vi "Apply Desired to Imported Data.vi"(0 "table.Data In":string[][](array[string]), 7 "StatArray":string[][](array[string]), 9 "Controller":T3, 11 "Stability Cluster":T4) -> (4 "table.Data Out":string[][](array[string]), 15 "StatBundle Out":T1(array[cluster]))   [LabVIEW 2013]
uses:
  TypeDef/Stability Cluster.ctl
  TypeDef/Controller Names.ctl
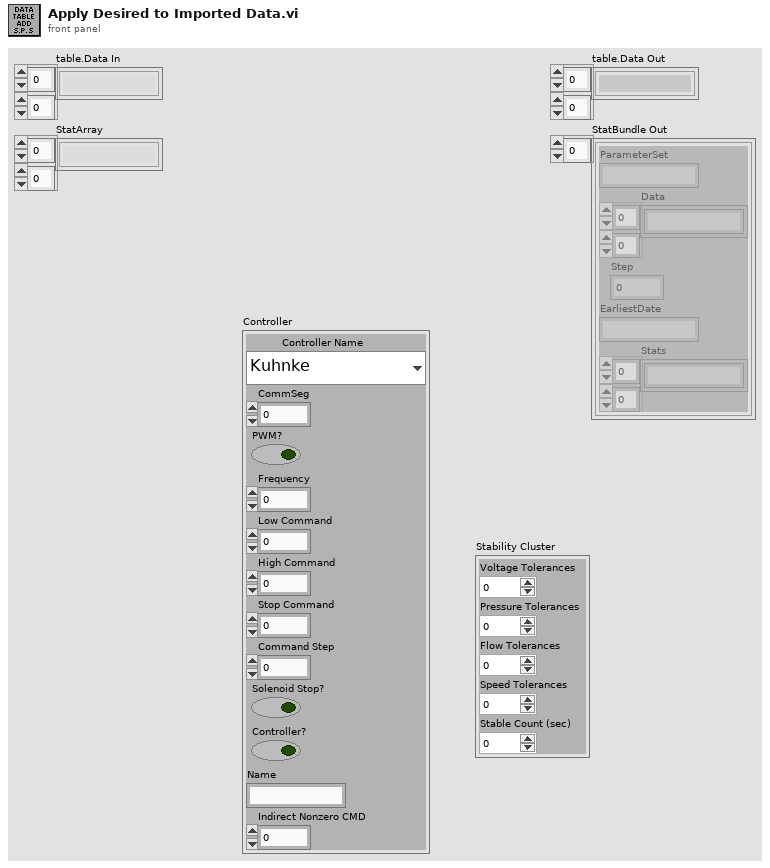
[diagram p1: front panel]
types:
  T1 = cluster{"ParameterSet":string, "Data":string[][], "Step":i32, "EarliestDate":string, "Stats":string[][]}[]
  T2 = typedef "Controller Names.ctl" = enum16{"Kuhnke", "McLaren", "Helbako BLDC", "Conti", "Hella E4LMF", "Hella E4LMD", "Hella E4DCG 20mm", "Hella E4DCG 30mm", "Helbako (old)", "TI PWM", "PSA", "Hella Hyundai Gas", "Hella Hyundai Diesel", "8 Comm", "10 Comm", "8 Comm Hella FCA", "10 Comm Hella FCA", "8 Comm Omron", "10 Comm Omron", "8 Comm Nissan", "10 Comm Nissan"}
  T3 = cluster{"Controller Name":T2, "CommSeg":i32, "PWM?":bool, "Frequency":i32, "Low Command":dbl, "High Command":dbl, "Stop Command":dbl, "Command Step":dbl, "Solenoid Stop?":bool, "Controller?":bool, "Name":string, "Indirect Nonzero CMD":dbl}
  T4 = typedef "Stability Cluster.ctl" = cluster{"Voltage Tolerances":dbl, "Pressure Tolerances":dbl, "Flow Tolerances":dbl, "Speed Tolerances":dbl, "Stable Count (sec)":dbl}
  T5 = typedef "Command Cluster.ctl" = cluster{"Para1":i32, "SP1":dbl, "Para2":i32, "SP2":dbl, "Para3":i32, "SP3":dbl}
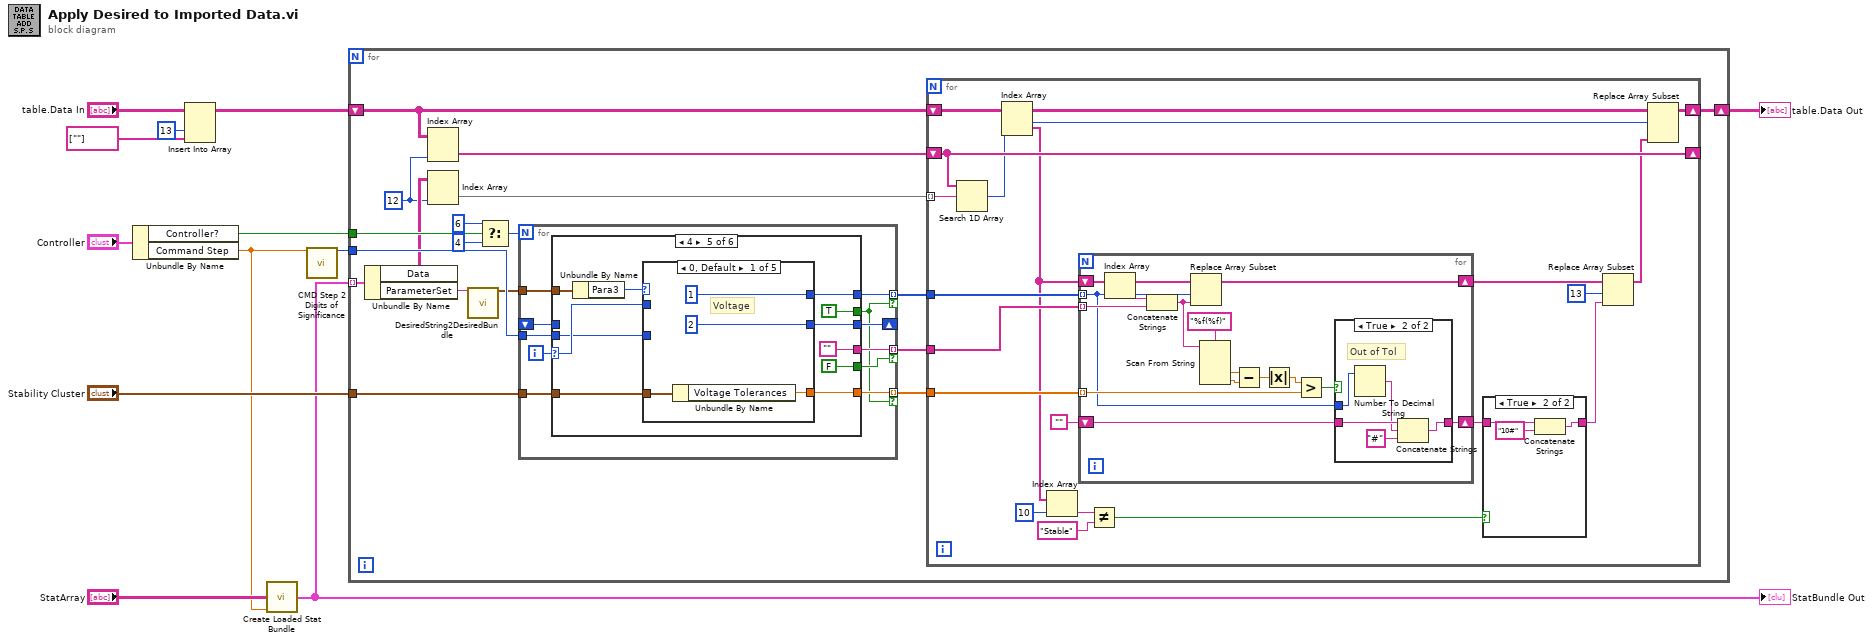
[diagram p0: block diagram]
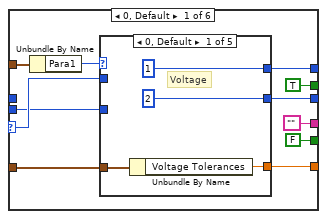
[diagram p4: hidden frame]
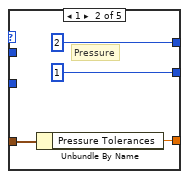
[diagram p5: hidden frame]
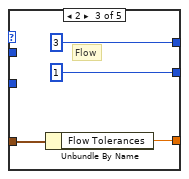
[diagram p6: hidden frame]
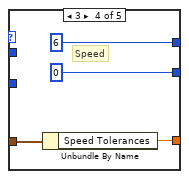
[diagram p7: hidden frame]
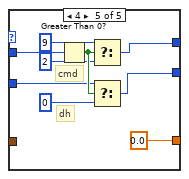
[diagram p8: hidden frame]
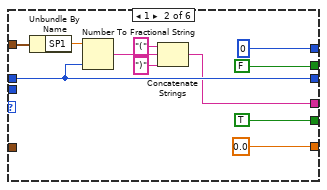
[diagram p9: hidden frame]
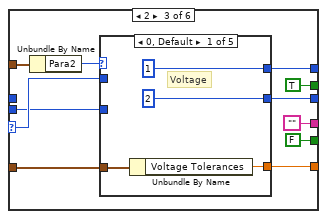
[diagram p10: hidden frame]
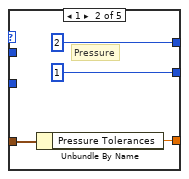
[diagram p11: hidden frame]
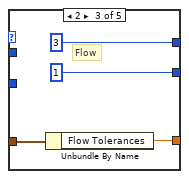
[diagram p12: hidden frame]
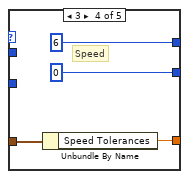
[diagram p13: hidden frame]
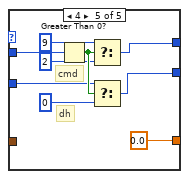
[diagram p14: hidden frame]
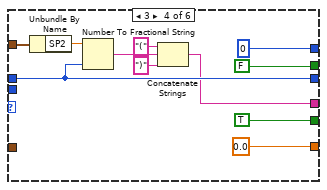
[diagram p15: hidden frame]
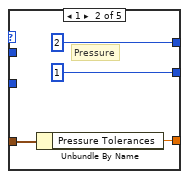
[diagram p16: hidden frame]
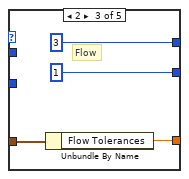
[diagram p17: hidden frame]
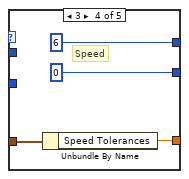
[diagram p18: hidden frame]
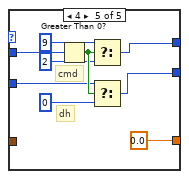
[diagram p19: hidden frame]
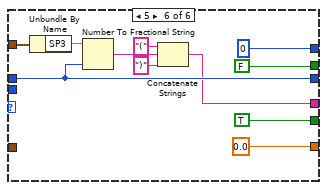
[diagram p20: hidden frame]
diagram:
  n1 = Unbundle By Name("Controller") -> ("Controller?"=w10:bool, "Command Step"=w1:dbl)
  n2 = Insert Into Array(array="table.Data In", index (col)=13 ("disabled index (col)"), new element=string[] [""]) -> (w4:string[][])  [unwired: 1 in]
  n3 = call "Create Loaded Stat Bundle.vi"("StatArray"="StatArray", "CMD Step"=w1) -> ("StatBundle Out"=w2:T1)  [unwired: 13 in]
  "StatBundle Out" <- w2
  n4 = call "CMD Step 2 Digits of Significance.vi"("CMD Step"=w1) -> ("Digits of Significance"=w11:i32)  [unwired: 14 in]
  n5 = for {
    tunnel: w2 -> [w30] mode=indexing
    tunnel: w11 -> [w25]
    tunnel: w10 -> [w24]
    tunnel: "Stability Cluster" -> [w22]
    shift-right: [w18] -> w8
    shift-left: w4 -> [w16]
    w14 = 12 ("disabled index (col)")
    n6 = Unbundle By Name(w30) -> ("Data"=w15:string[][], "ParameterSet"=w29:string)
    n7 = Index Array(array=w16, index (col)=w14) -> (element=w13:string[])  [unwired: 1 in]
    n8 = Index Array(array=w15, index (col)=w14) -> (element=w17:string[])  [unwired: 1 in]
    n9 = call "DesiredString2DesiredBundle.vi"("ParameterSet"=w29) -> ("DesiredParameters"=w23:T5)  [unwired: 13 in, 1 out]
    n10 = Select(t=6, s=w24, f=4) -> (s? t:f=w26:i32)
    n11 = for {
      N: w26 -> [_]
      tunnel: w23 -> [w84]
      shift-right: [w82] -> _
      shift-left: _ -> [w81]
      tunnel: [w83] -> w19 mode=indexing if=w76
      tunnel: [w80] -> w20 mode=indexing if=w79
      tunnel: w22 -> [w78]
      tunnel: [w77] -> w21 mode=indexing if=w76
      tunnel: w25 -> [w75]
      i -> [w85]
      n12 = case shown="4" w85 {
        selector: w85 -> [w94 _ w138 _ w182 _]
        tunnel: w84 -> [w96 w132 w143 w179 w190 w226]
        tunnel: [w93 0 w135 0 w186 0] -> w83
        tunnel: [w92 w129 w134 w176 w185 w223] -> w82
        tunnel: w81 -> [_ w129 _ w176 _ w223]
        tunnel: ["" w126 "" w175 "" w220] -> w80
        tunnel: [TRUE FALSE TRUE FALSE TRUE FALSE] -> w76
        tunnel: [FALSE TRUE FALSE TRUE FALSE TRUE] -> w79
        tunnel: w78 -> [w88 _ w137 _ w183 _]
        tunnel: [w87 0.0 ("Speed Tolerances") w136 0.0 ("Speed Tolerances") w184 0.0 ("Speed Tolerances")] -> w77
        tunnel: w75 -> [w86 _ w133 _ w180 _]
        frame 0, Default {
          n13 = Unbundle By Name(w96) -> ("Para1"=w95:i32)
          n14 = case shown="0, Default" w95 {
            tunnel: [1 2 3 6 w120] -> w93
            tunnel: w94 -> [_ _ _ _ w121]
            tunnel: [2 1 1 0 w117] -> w92
            tunnel: w88 -> [w98 w102 w106 w110 _]
            tunnel: [w97 w101 w105 w109 0.0 ("Speed Tolerances")] -> w87
            tunnel: w86 -> [_ _ _ _ w113]
            frame 0, Default {
              # "Voltage"
              n15 = Unbundle By Name(w98) -> ("Voltage Tolerances"=w97:dbl)
            }
            frame 1 {
              # "Pressure"
              n16 = Unbundle By Name(w102) -> ("Pressure Tolerances"=w101:dbl)
            }
            frame 2 {
              # "Flow"
              n17 = Unbundle By Name(w106) -> ("Flow Tolerances"=w105:dbl)
            }
            frame 3 {
              # "Speed"
              n18 = Unbundle By Name(w110) -> ("Speed Tolerances"=w109:dbl)
            }
            frame 4 {
              # "dh"
              # "cmd"
              n19 = Greater Than 0?(x=w121) -> (x > 0?=w118:bool)
              n20 = Select(t=9, s=w118, f=2) -> (s? t:f=w120:i32)
              n21 = Select(t=w113, s=w118, f=0) -> (s? t:f=w117:i32)
            }
          }
        }
        frame 1 {
          n22 = Unbundle By Name(w132) -> ("SP1"=w131:dbl)
          n23 = Number To Fractional String(number=w131, precision (6)=w129) -> (F-format string=w130:string)  [unwired: 2 in]
          n24 = Concatenate Strings("(" ("string"), w130, ")" ("string")) -> (w126:string)
        }
        frame 2 {
          n25 = Unbundle By Name(w143) -> ("Para2"=w139:i32)
          n26 = case shown="0, Default" w139 {
            tunnel: [1 2 3 6 w167] -> w135
            tunnel: w138 -> [_ _ _ _ w168]
            tunnel: [2 1 1 0 w164] -> w134
            tunnel: w137 -> [w145 w149 w153 w157 _]
            tunnel: [w144 w148 w152 w156 0.0 ("Speed Tolerances")] -> w136
            tunnel: w133 -> [_ _ _ _ w160]
            frame 0, Default {
              # "Voltage"
              n27 = Unbundle By Name(w145) -> ("Voltage Tolerances"=w144:dbl)
            }
            frame 1 {
              # "Pressure"
              n28 = Unbundle By Name(w149) -> ("Pressure Tolerances"=w148:dbl)
            }
            frame 2 {
              # "Flow"
              n29 = Unbundle By Name(w153) -> ("Flow Tolerances"=w152:dbl)
            }
            frame 3 {
              # "Speed"
              n30 = Unbundle By Name(w157) -> ("Speed Tolerances"=w156:dbl)
            }
            frame 4 {
              # "dh"
              # "cmd"
              n31 = Greater Than 0?(x=w168) -> (x > 0?=w165:bool)
              n32 = Select(t=9, s=w165, f=2) -> (s? t:f=w167:i32)
              n33 = Select(t=w160, s=w165, f=0) -> (s? t:f=w164:i32)
            }
          }
        }
        frame 3 {
          n34 = Unbundle By Name(w179) -> ("SP2"=w178:dbl)
          n35 = Number To Fractional String(number=w178, precision (6)=w176) -> (F-format string=w177:string)  [unwired: 2 in]
          n36 = Concatenate Strings("(" ("string"), w177, ")" ("string")) -> (w175:string)
        }
        frame 4 {
          n37 = Unbundle By Name(w190) -> ("Para3"=w181:i32)
          n38 = case shown="0, Default" w181 {
            tunnel: [1 2 3 6 w214] -> w186
            tunnel: w182 -> [_ _ _ _ w215]
            tunnel: [2 1 1 0 w211] -> w185
            tunnel: w183 -> [w192 w196 w200 w204 _]
            tunnel: [w191 w195 w199 w203 0.0 ("Speed Tolerances")] -> w184
            tunnel: w180 -> [_ _ _ _ w207]
            frame 0, Default {
              # "Voltage"
              n39 = Unbundle By Name(w192) -> ("Voltage Tolerances"=w191:dbl)
            }
            frame 1 {
              # "Pressure"
              n40 = Unbundle By Name(w196) -> ("Pressure Tolerances"=w195:dbl)
            }
            frame 2 {
              # "Flow"
              n41 = Unbundle By Name(w200) -> ("Flow Tolerances"=w199:dbl)
            }
            frame 3 {
              # "Speed"
              n42 = Unbundle By Name(w204) -> ("Speed Tolerances"=w203:dbl)
            }
            frame 4 {
              # "dh"
              # "cmd"
              n43 = Greater Than 0?(x=w215) -> (x > 0?=w212:bool)
              n44 = Select(t=9, s=w212, f=2) -> (s? t:f=w214:i32)
              n45 = Select(t=w207, s=w212, f=0) -> (s? t:f=w211:i32)
            }
          }
        }
        frame 5 {
          n46 = Unbundle By Name(w226) -> ("SP3"=w225:dbl)
          n47 = Number To Fractional String(number=w225, precision (6)=w223) -> (F-format string=w224:string)  [unwired: 2 in]
          n48 = Concatenate Strings("(" ("string"), w224, ")" ("string")) -> (w220:string)
        }
      }
    }
    n49 = for {
      tunnel: w21 -> [w47]
      tunnel: w20 -> [w46]
      tunnel: w19 -> [w45]
      shift-right: [w39] -> w18
      shift-left: w16 -> [w40]
      tunnel: w17 -> [w37] mode=indexing
      shift-right: [w38] -> _
      shift-left: w13 -> [w38]
      n50 = Search 1D Array(1D array=w38, element=w37) -> (index of element=w36:i32)  [unwired: 1 in]
      n51 = Index Array(array=w40, index (row)=w36) -> (element=w35:string[])  [unwired: 1 in]
      n52 = Index Array(array=w35, index=10) -> (element=w43:string)
      n53 = for {
        shift-right: [w67] -> w34
        shift-left: w35 -> [w68]
        tunnel: w45 -> [w54] mode=indexing
        tunnel: w46 -> [w65] mode=indexing
        tunnel: w47 -> [w58] mode=indexing
        shift-right: [w55] -> w48
        shift-left: "" -> [w56]
        n54 = Index Array(array=w68, index=w54) -> (element=w66:string)
        n55 = Concatenate Strings(w66, w65) -> (w63:string)
        n56 = Replace Array Subset(array=w68, new element=w63, index=w54) -> (w67:string[])
        n57 = Scan From String(format string="%f(%f)", input string=w63) -> (output 1=w62:dbl, output 2=w61:dbl)  [unwired: 4 in, 3 out]
        n58 = Subtract(x=w62, y=w61) -> (x-y=w60:dbl)
        n59 = Absolute Value(x=w60) -> (abs(x)=w59:dbl)
        n60 = Greater?(x=w59, y=w58) -> (0:w57:bool)
        n61 = case shown="True" w57 {
          tunnel: [w69 w70] -> w55
          tunnel: w56 -> [w69 w73]
          tunnel: w54 -> [_ w74]
          frame False {
            # "In Tol"
          }
          frame True {
            # "Out of Tol"
            n62 = Number To Decimal String(number=w74) -> (decimal integer string=w72:string)  [unwired: 1 in]
            n63 = Concatenate Strings(w73, w72, "#" ("string")) -> (w70:string)
          }
        }
      }
      n64 = Not Equal?(x=w43, y="Stable") -> (x != y?=w41:bool)
      n65 = case shown="True" w41 {
        tunnel: w48 -> [w50 w52]
        tunnel: [w50 w51] -> w33
        frame False {
        }
        frame True {
          n66 = Concatenate Strings(w52, "10#" ("string")) -> (w51:string)
        }
      }
      n67 = Replace Array Subset(array=w34, new element=w33, index=13) -> (w31:string[])
      n68 = Replace Array Subset(array=w40, new element=w31, index (row)=w36) -> (w39:string[][])  [unwired: 1 in]
    }
  }
  "table.Data Out" <- w8
